vi "ROI group interface 2.vi"(8 "error in (no error)":errorcluster) -> (0 "error out":errorcluster)   [LabVIEW 2017]
panel:
  out "POI on selected plane":dbl[][](array[numeric])
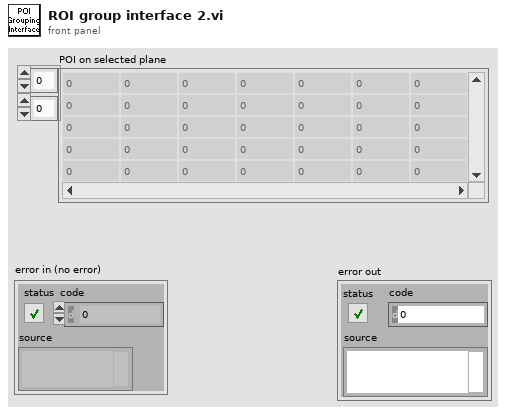
[diagram p1: front panel]
types:
  T1 = typedef "Image Type" = u32
  T2 = enum32{"Invalid", "Standard", "Closed", "Hidden", "Minimized", "Maximized"}
  T3 = typedef "IMAQ Image.ctl" = refnum<image>
  T4 = typedef "ROI Descriptor" = cluster{"Global Rectangle":i32[], "Contours":cluster{"ID":enum32{"External", "Internal"}, "Type":u32, "Coordinates":i32[]}[]}
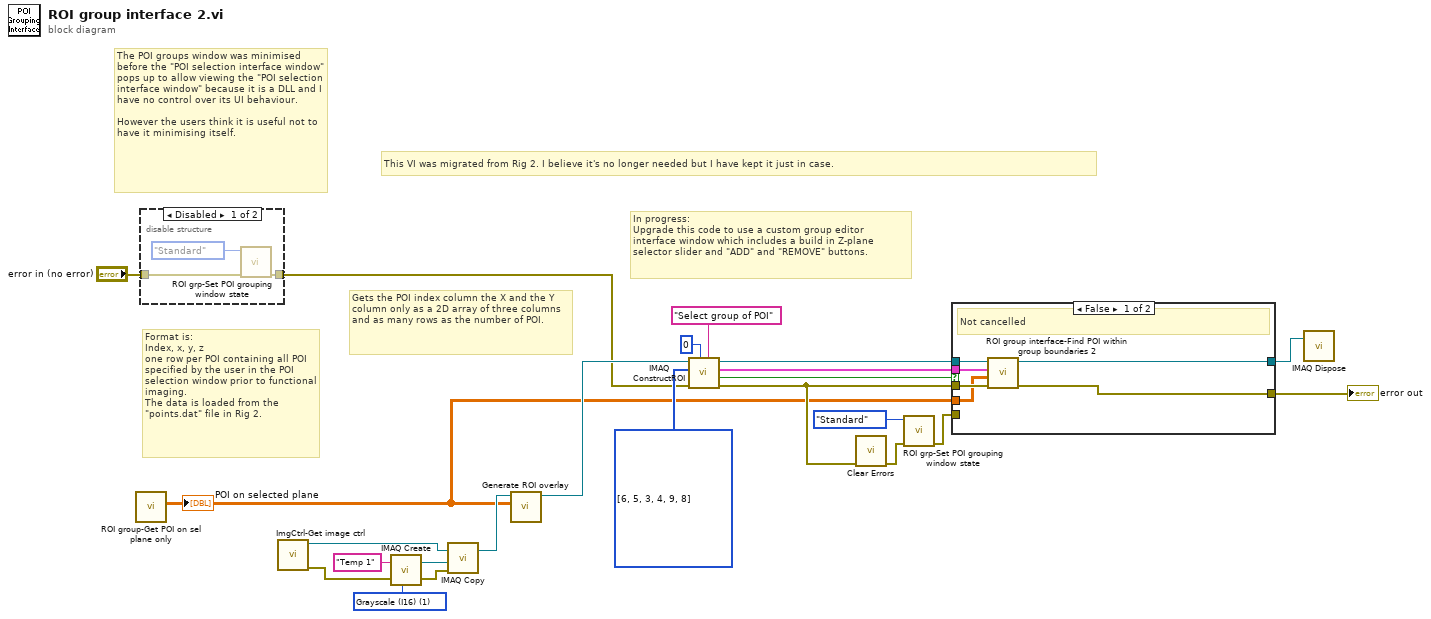
[diagram p0: block diagram]
diagram:
  w8 = T1 1 items=["Grayscale (U8)", "Grayscale (I16)", "Grayscale (SGL)", "Complex (CSG)", "RGB (U32)", "HSL (U32)", "RGB (U64)", "Grayscale (U16)"] ("Image Type")
  w22 = u32[] [6, 5, 3, 4, 9, 8] items=["No Selection", "Point", "Line", "Rectangle", "Oval", "Polygon", "Freehand Region", "Annulus", "Zoom", "Pan", "Broken Line", "Freehand Line", "Rotated Rectangle"] ("Tools")
  # "This VI was migrated from Rig 2. I believe it's no longer needed but I have kept it just in case."
  # "Gets the POI index column the X and the Y column only as a 2D array of three columns and as many rows as the number of POI."
  # "Format is: \nIndex, x, y, z\none row per POI containing all POI specified by the user in the POI selection window prior to functional imaging.\nThe data is loaded from the \"points.dat\" file in Rig 2."
  # "The POI groups window was minimised before the \"POI selection interface window\" pops up to allow viewing the \"POI selection interface window\" because it is a DLL and I have no control over its UI behaviour.\n\nHowever the users think it is useful not to have it minimising itself."
  # "In progress:\nUpgrade this code to use a custom group editor interface window which includes a build in Z-plane selector slider and \"ADD\" and \"REMOVE\" buttons."
  n1 = call "ROI group-Get POI on sel plane only.vi"() -> ("POI on selected plane"=w5:dbl[][])  [unwired: 11 in]
  "POI on selected plane" <- w5
  n2 = disable-structure shown="Disabled" {
    disable-tunnel: "error in (no error)" -> [w25 w27]
    disable-tunnel: [w24 w27] -> w15
    frame Disabled {
      n3 = call "ROI grp-Set POI grouping window state.vi"("error in (no error)"=w25, "Front Panel Window:State"=T2."Standard") -> ("error out"=w24:errorcluster)  [unwired: 9 in]
    }
    frame Enabled {
    }
  }
  n4 = call "ImgCtrl-Get image ctrl.vi"() -> ("error out"=w3:errorcluster, "Image"=w4:T3)  [unwired: 10 in]
  n5 = call "IMAQ Create"("Image Name"="Temp 1", "Image Type"=w8, "error in (no error)"=w3) -> ("New Image"=w7:T3, "error out"=w2:errorcluster)  [unwired: 2 in]
  n6 = call "IMAQ Copy"("error in (no error)"=w2, "Image Dst"=w7, "Image Src"=w4) -> ("Image Dst Out"=w6:T3)  [unwired: 3 in, 1 out]
  n7 = call "Generate ROI overlay.vi"("POI on selected plane"=w5, "Refnum in"=w6) -> ("Refnum out"=w20:T3)  [unwired: 9 in]
  n8 = call "IMAQ ConstructROI"("Prompt"="Select group of POI", "Window Number (-1...15)"=0, "error in (no error)"=w15, "Tools"=w22, "Image"=w20) -> ("error out"=w12:errorcluster, "Cancel"=w17:bool, "ROI Descriptor Out"=w18:T4, "Image Out (duplicate)"=w19:T3)  [unwired: 3 in]
  n9 = call <vilib>:"Clear Errors.vi"("error in (no error)"=w12) -> ("error out"=w13:errorcluster)  [unwired: 5 in, 1 out]
  n10 = call "ROI grp-Set POI grouping window state.vi"("error in (no error)"=w13, "Front Panel Window:State"=T2."Standard") -> ("error out"=w11:errorcluster)  [unwired: 9 in]
  n11 = case shown="False" w17 {
    tunnel: w19 -> [w33 w35]
    tunnel: w12 -> [w32 w34]
    tunnel: w18 -> [w29 _]
    tunnel: w5 -> [w31 _]
    tunnel: [w30 w35] -> w10
    tunnel: [w28 w34] -> w1
    tunnel: w11 -> [_ _]
    frame False {
      # "Not cancelled"
      n12 = call "ROI group interface-Find POI within group boundaries 2.vi"("error in (no error)"=w32, "X-Y coordinates array of POI"=w31, "ROI Descriptor Out"=w29, "Image ref in"=w33) -> ("error out"=w28:errorcluster, "Image ref shift out"=w30:T3)  [unwired: 4 in, 2 out]
    }
    frame True {
      # "Cancelled"
    }
  }
  "error out" <- w1
  n13 = call "IMAQ Dispose"("Image"=w10) -> ()  [unwired: 5 in, 1 out]
